vi "Write enable rmb user.vi"(8 "error in (no error)":errorcluster, 10 "enable rmb user":bool, 11 "[V] Login in":refnum<class "[V] Login.lvclass">) -> (0 "error out":errorcluster, 3 "[V] Login out":refnum<class "[V] Login.lvclass">)   [LabVIEW 2020, in "[V] Login.lvlib" / "[V] Login.lvclass"]
uses:
  [V] Login.lvclass
  [V] Login.lvclass/[V] Login.ctl
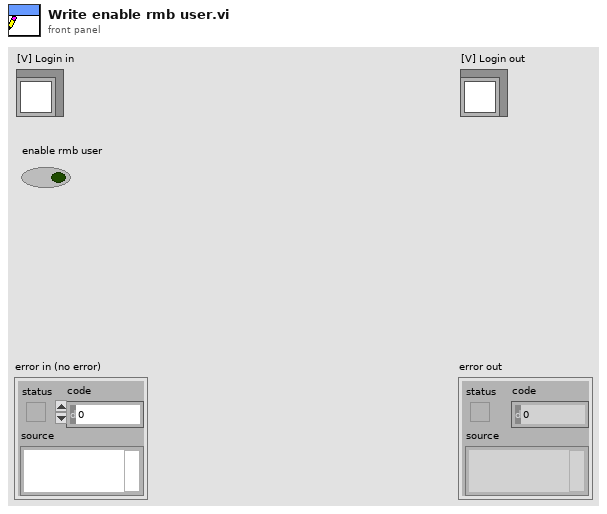
[diagram p1: front panel]
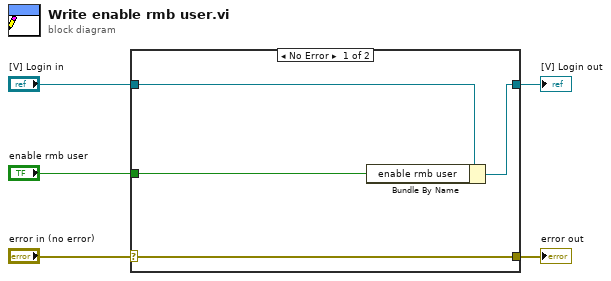
[diagram p0: block diagram]
diagram:
  n1 = case shown="No Error" "error in (no error)" {
    selector: "error in (no error)" -> [w9 w10]
    tunnel: [w9 w10] -> w4
    tunnel: [w7 w11] -> w2
    tunnel: "[V] Login in" -> [w8 w11]
    tunnel: "enable rmb user" -> [w6 _]
    frame No Error {
      n2 = Bundle By Name(cluster=w8, "enable rmb user"=w6) -> (w7:refnum<class "[V] Login.lvclass">)
    }
    frame Error {
    }
  }
  "error out" <- w4
  "[V] Login out" <- w2
